vi "Load Material Theme.vi"(11 "file path":path) -> (0 "error out":errorcluster, 1 "text":string, 2 "Theme":refnum<class "Material Theme.lvclass">)   [LabVIEW 2021, in "TSC Material Theme.lvlib" / "Material Theme.lvclass"]
doc: "Load a material theme from disk in a JSON file format.\n\n<b>Note</b>: legacy XML files from version <v4 can still be loaded with this VI but should not be saved going forward.\n\n<b>Code Developed By:</b>\nTechnology Service Corporation\nwww.tsc.com/atcs\n\nDeveloper:\nDaniel Coons"
uses:
  Material Theme.lvclass
  Material Theme.lvclass/Material Theme.ctl
  <vilib>/JDP Science/JSONtext/LVClass Serializer/JSONtext LVClass Serializer.lvclass
  Material-Scheme/Material-Scheme.lvclass
  Material-Palette/Material-Palette.lvclass
  <vilib>/JDP Science/JSONtext/JSONtext.lvlib
  30a1bc54-b62a-49a8-8efc-2c13e9e1dba8.vi
  3cd4fc15-787d-41cf-acd3-45f4c7af28a3.vi
  8d0b8e92-f2d2-4725-af73-822fbd61956a.vi
  TSC Material Theme.lvlib
panel:
  # "FOR DEBUG"
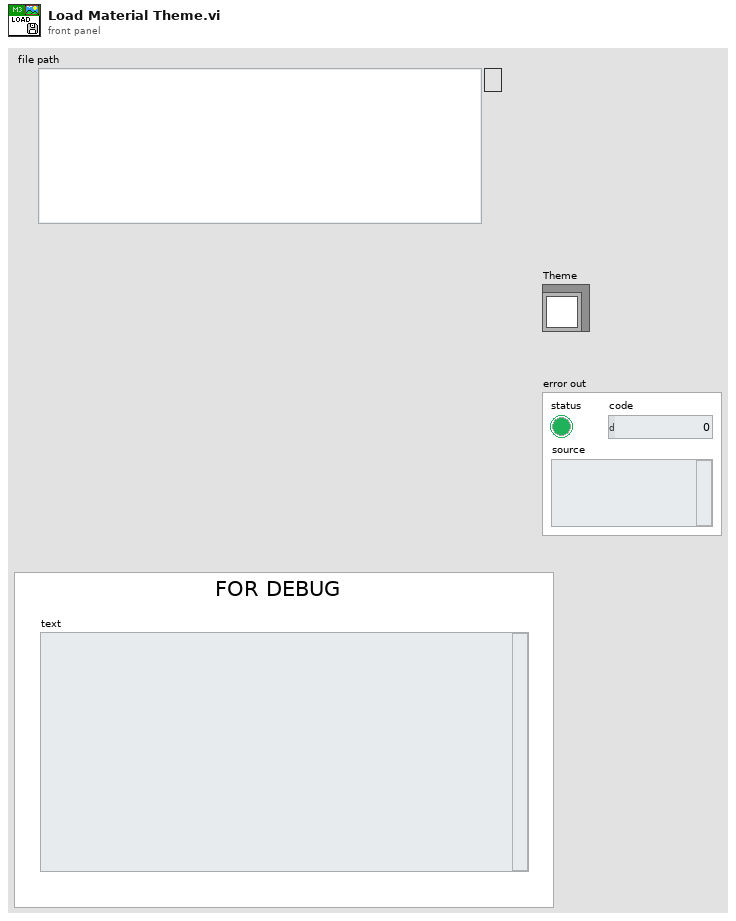
[diagram p1: front panel]
types:
  T1 = cluster{"primary":u32, "secondary":u32, "tertiary":u32, "error":u32}
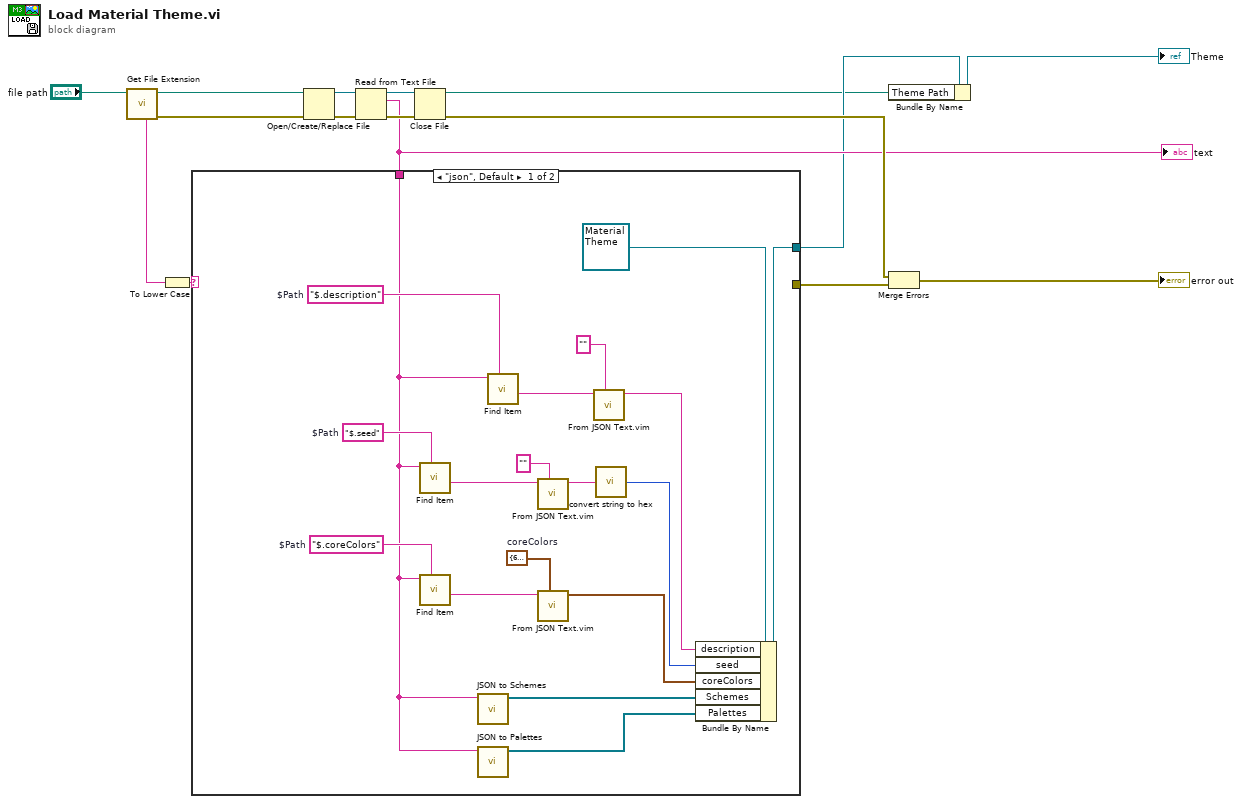
[diagram p0: block diagram]
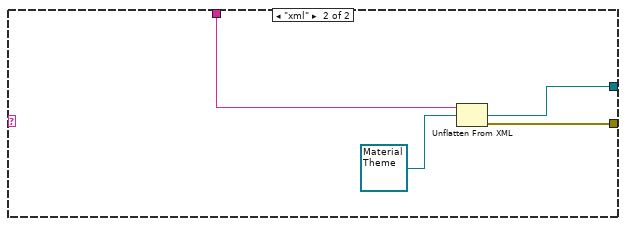
[diagram p2: hidden frame]
diagram:
  n1 = call <vilib>:"Get File Extension.vi"("file"="file path") -> ("error out"=w11:errorcluster, "dup file"=w3:path, "unmodified file extension"=w2:string)  [unwired: 6 in, 2 out]
  n2 = To Lower Case(string=w2) -> (all lower case string=w1:string)
  n3 = Open/Create/Replace File(file path (use dialog)=w3, error in=w11) -> (refnum out=w10:refnum<file>, error out=w16:errorcluster)  [unwired: 4 in, 1 out]
  n4 = Read from Text File(file (use dialog)=w10, error in=w16) -> (refnum out=w9:refnum<file>, text=w8:string, error out=w15:errorcluster)  [unwired: 2 in, 1 out]
  "text" <- w8
  n5 = case shown="\"json\", Default" w1 {
    tunnel: [_ w38] -> w12
    tunnel: w8 -> [w20 w37]
    tunnel: [w33 w35] -> w6
    frame "json", Default {
      w21 = "$.coreColors"  # $Path
      w18 = T1 {"primary"=6641039, "secondary"=6445937, "tertiary"=8213088, "error"=11740702}  # coreColors
      w28 = "$.seed"  # $Path
      w30 = "$.description"  # $Path
      n6 = call <vilib>:"Find Item.vi"("$Path or Item Name"=w28, "JSON"=w20) -> ("<JSON>"=w26:string)  [unwired: 6 in, 3 out]
      n7 = call <vilib>:"Find Item.vi"("$Path or Item Name"=w21, "JSON"=w20) -> ("<JSON>"=w19:string)  [unwired: 6 in, 3 out]
      n8 = call "JSON to Schemes.vi"("Material JSON"=w20) -> ("Schemes"=w22:refnum<class "Material-Scheme.lvclass">[])  [unwired: 9 in, 1 out]
      n9 = call "JSON to Palettes.vi"("Material JSON"=w20) -> ("Palettes"=w23:refnum<class "Material-Palette.lvclass">[])  [unwired: 9 in, 1 out]
      n10 = call <vilib>:"Find Item.vi"("$Path or Item Name"=w30, "JSON"=w20) -> ("<JSON>"=w32:string)  [unwired: 6 in, 3 out]
      n11 = call "From JSON Text.vim"("Data Type and Default Value"="", "JSON"=w26) -> ("Data out"=w25:string)  [unwired: 8 in, 1 out]
      n12 = call "From JSON Text.vim"("Data Type and Default Value"=w18, "JSON"=w19) -> ("Data out"=w17:T1)  [unwired: 8 in, 1 out]
      n13 = call "From JSON Text.vim"("Data Type and Default Value"="", "JSON"=w32) -> ("Data out"=w29:string)  [unwired: 8 in, 1 out]
      n14 = call "convert string to hex.vi"("string"=w25) -> ("hex"=w24:u32)
      n15 = Bundle By Name(cluster=refnum<class "Material Theme.lvclass"> refnum ("output cluster"), "description"=w29, "seed"=w24, "coreColors"=w17, "Schemes"=w22, "Palettes"=w23) -> (w33:refnum<class "Material Theme.lvclass">)
    }
    frame "xml" {
      n16 = Unflatten From XML(xml string=w37, type=refnum<class "Material Theme.lvclass"> refnum ("output cluster")) -> (value=w35:refnum<class "Material Theme.lvclass">, error out=w38:errorcluster)  [unwired: 1 in]
    }
  }
  n17 = Close File(refnum=w9, error in=w15) -> (path=w4:path, error out=w14:errorcluster)
  n18 = Bundle By Name(cluster=w6, "Theme Path"=w4) -> (→"Theme":refnum<class "Material Theme.lvclass">)
  n19 = Merge Errors(w14, w12) -> (→"error out":errorcluster)
